vi "float_switch_check_debug.vi"(0 "Temperature Refnum":refnum<vi>, 1 "Heater Refnum":refnum<vi>, 2 "Abs Pressure Refnum":refnum<vi>, 3 "Abs Temperature Limit Refnum":refnum<vi>, 4 "Timeout Refnum":refnum<vi>, 5 "Abs Pressure Limit Refnum":refnum<vi>, 6 "STOP! Refnum":refnum<vi>, 7 "Pulse Generator Slide Refnum":refnum<vi>, 8 "Float Indicator Refnum":refnum<vi>[](array[refnum]), 9 "lines":tag[](array[tag])) -> ()   [LabVIEW 2015]
uses:
  <vilib>/DAQmx/create/channels.llb/DAQmx Create Channel (DI-Digital Input).vi
  <vilib>/DAQmx/read.llb/DAQmx Read (Digital 1D Bool NChan 1Samp 1Line).vi
panel:
  out "Stopwatch Elapsed":dbl
  out "Stopwatch Start":dbl
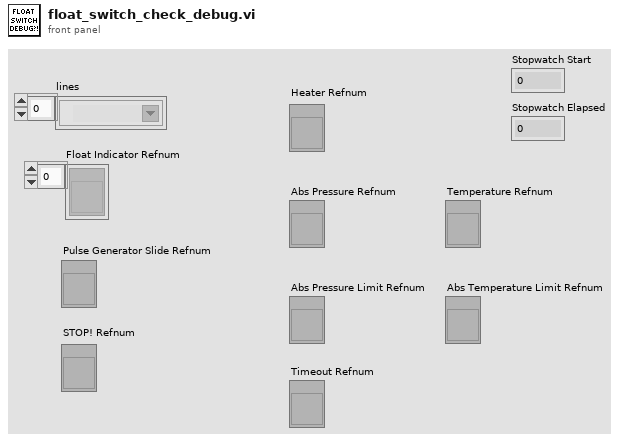
[diagram p1: front panel]
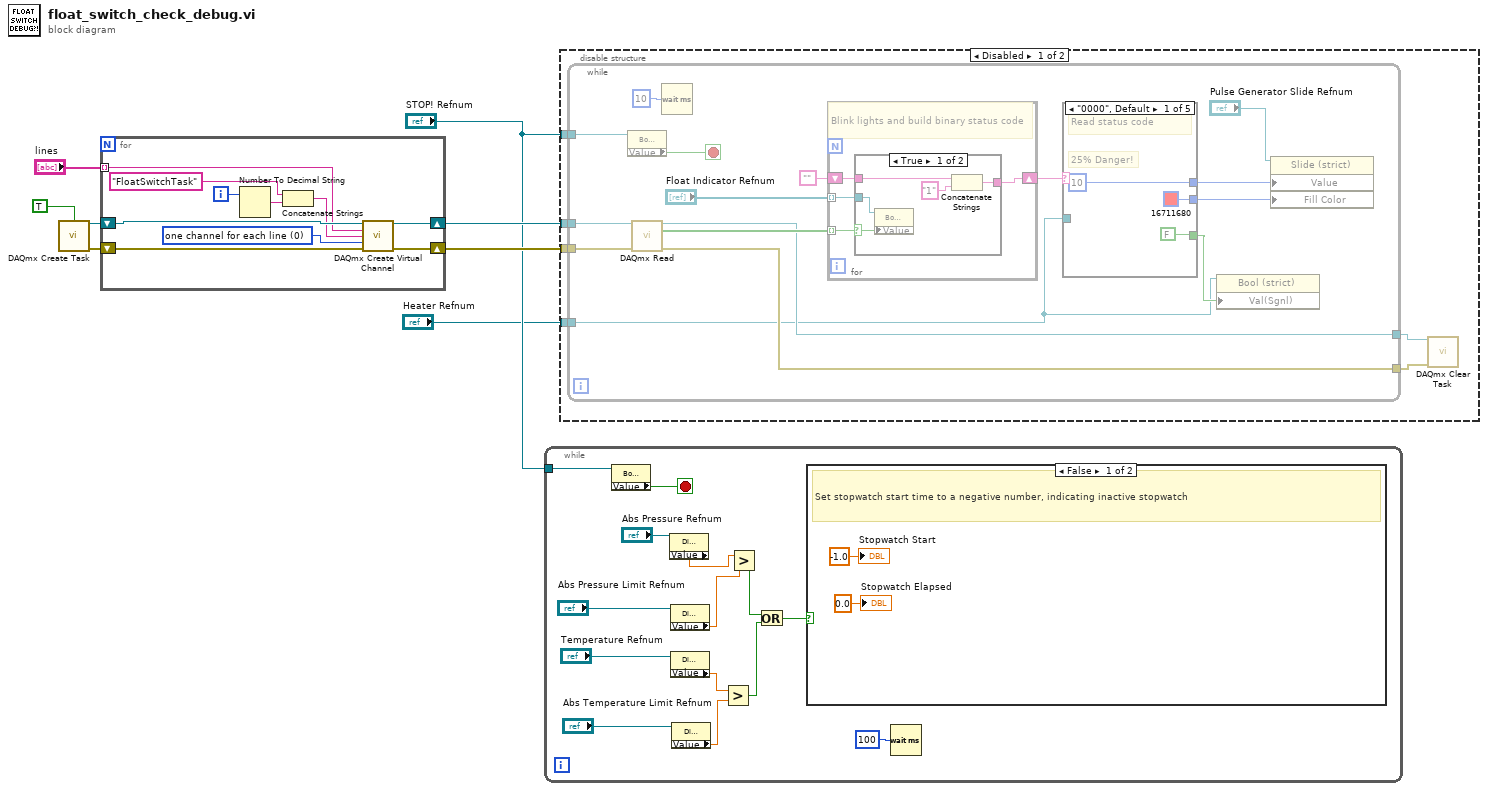
[diagram p0: block diagram]
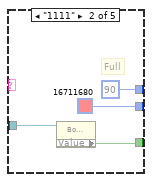
[diagram p2: hidden frame]
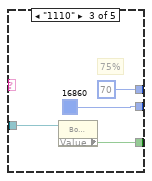
[diagram p3: hidden frame]
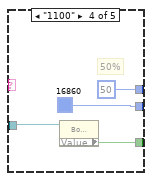
[diagram p4: hidden frame]
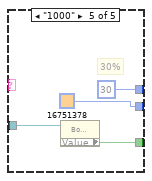
[diagram p5: hidden frame]
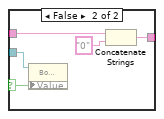
[diagram p6: hidden frame]
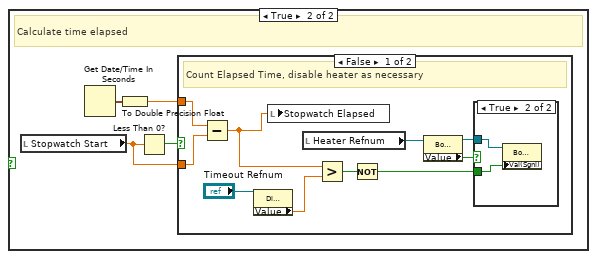
[diagram p8: hidden frame]
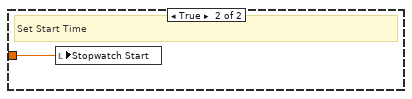
[diagram p10: hidden frame]
diagram:
  n1 = call <vilib>:"DAQmx Create Task.vi"("auto cleanup"=TRUE) -> ("task out"=w7:refnum<k21>, "error out"=w6:errorcluster)  [unwired: 13 in]
  n2 = for {
    shift-right: [w18] -> w5
    shift-left: w7 -> [w16]
    shift-right: [w17] -> w4
    shift-left: w6 -> [w15]
    tunnel: "lines" -> [w14] mode=indexing
    i -> [w9]
    w11 = 0 items=["one channel for each line", "one channel for all lines"] ("line grouping")
    n3 = Number To Decimal String(number=w9) -> (decimal integer string=w12:string)  [unwired: 1 in]
    n4 = Concatenate Strings("FloatSwitchTask" ("string"), w12) -> (w10:string)
    n5 = call-poly <vilib>:"DAQmx Create Virtual Channel.vi"("task in"=w16, "lines"=w14, "name to assign"=w10, "line grouping"=w11, "error in"=w15) -> ("task out"=w18:refnum<k21>, "error out"=w17:errorcluster)  [unwired: 9 in]
  }
  n6 = while {
    tunnel: "STOP! Refnum" -> [w31]
    stop <- w32 stop-if-true
    n7 = property class="Bool (strict)"(reference=w31) -> ("Value"=w32:bool)  [unwired: 1 in, 2 out]
    n8 = property class="DigNum (strict)"(reference="Abs Pressure Refnum") -> ("Value"=w20:dbl)  [unwired: 1 in, 2 out]
    n9 = property class="DigNum (strict)"(reference="Abs Pressure Limit Refnum") -> ("Value"=w19:dbl)  [unwired: 1 in, 2 out]
    n10 = property class="DigNum (strict)"(reference="Temperature Refnum") -> ("Value"=w25:dbl)  [unwired: 1 in, 2 out]
    n11 = property class="DigNum (strict)"(reference="Abs Temperature Limit Refnum") -> ("Value"=w24:dbl)  [unwired: 1 in, 2 out]
    n12 = Greater?(x=w25, y=w24) -> (0:w22:bool)
    n13 = Greater?(x=w20, y=w19) -> (0:w23:bool)
    n14 = Or(x=w23, y=w22) -> (x .or. y?=w21:bool)
    n15 = case shown="False" w21 {
      frame False {
        # "Set stopwatch start time to a negative number, indicating inactive stopwatch"
        "Stopwatch Start" <- -1.0 ("Stopwatch Start")
        "Stopwatch Elapsed" <- 0.0 ("Stopwatch Elapsed")
      }
      frame True {
        # "Calculate time elapsed"
        n16 = local read "Stopwatch Start"() -> (w35:dbl)
        n17 = Get Date/Time In Seconds() -> (seconds since 1Jan1904=w37:timestamp)
        n18 = To Double Precision Float(number=w37) -> (double precision float=w36:dbl)
        n19 = Less Than 0?(x=w35) -> (x < 0?=w38:bool)
        n20 = case shown="False" w38 {
          tunnel: w36 -> [w48 w51]
          tunnel: w35 -> [w47 _]
          frame False {
            # "Count Elapsed Time, disable heater as necessary"
            n21 = Subtract(x=w48, y=w47) -> (x-y=w43:dbl)
            n22 = property class="DigNum (strict)"(reference="Timeout Refnum") -> ("Value"=w45:dbl)  [unwired: 1 in, 2 out]
            n23 = local write "Stopwatch Elapsed"(w43) -> ()
            n24 = local read "Heater Refnum"() -> (w42:refnum<vi>)
            n25 = Greater?(x=w43, y=w45) -> (0:w44:bool)
            n26 = Not(x=w44) -> (.not. x?=w39:bool)
            n27 = property class="Bool (strict)"(reference=w42) -> (reference out=w40:refnum<vi>, "Value"=w41:bool)  [unwired: 1 in, 1 out]
            n28 = case shown="True" w41 {
              tunnel: w40 -> [_ w50]
              tunnel: w39 -> [_ w49]
              frame False {
              }
              frame True {
                n29 = property class="Bool (strict)"(reference=w50, "Val(Sgnl)"=w49) -> ()  [unwired: 1 in, 2 out]
              }
            }
          }
          frame True {
            # "Set Start Time"
            n30 = local write "Stopwatch Start"(w51) -> ()
          }
        }
      }
    }
    n31 = Wait (ms)(milliseconds to wait=u32 100) -> ()  [unwired: 1 out]
  }
  n32 = disable-structure shown="Disabled" {
    disable-tunnel: w5 -> [w57 _]
    disable-tunnel: w4 -> [w56 _]
    disable-tunnel: "STOP! Refnum" -> [w53 _]
    disable-tunnel: "Heater Refnum" -> [w52 _]
    frame Disabled {
      n33 = while {
        tunnel: w57 -> [w68]
        tunnel: w56 -> [w67]
        tunnel: w53 -> [w63]
        tunnel: [w60] -> w55
        tunnel: [w59] -> w54
        tunnel: w52 -> [w58]
        stop <- w62 stop-if-true
        n34 = property class="Bool (strict)"(reference=w63) -> ("Value"=w62:bool)  [unwired: 1 in, 2 out]
        n35 = call-poly <vilib>:"DAQmx Read.vi"("task/channels in"=w68, "error in"=w67) -> ("task out"=w60:refnum<k21>, "data"=w73:bool[], "error out"=w59:errorcluster)  [unwired: 11 in]
        n36 = Wait (ms)(milliseconds to wait=u32 10) -> ()  [unwired: 1 out]
        n37 = for {
          tunnel: w73 -> [w96] mode=indexing
          tunnel: "Float Indicator Refnum" -> [w95] mode=indexing
          shift-right: [w93] -> w71
          shift-left: "" -> [w94]
          # "Blink lights and build binary status code"
          n38 = case shown="True" w96 {
            selector: w96 -> [w100 w105]
            tunnel: w95 -> [w101 w106]
            tunnel: w94 -> [w99 w103]
            tunnel: [w97 w102] -> w93
            frame True {
              n39 = property class="Bool (strict)"(reference=w101, "Value"=w100) -> ()  [unwired: 1 in, 2 out]
              n40 = Concatenate Strings(w99, "1" ("string")) -> (w97:string)
            }
            frame False {
              n41 = property class="Bool (strict)"(reference=w106, "Value"=w105) -> ()  [unwired: 1 in, 2 out]
              n42 = Concatenate Strings(w103, "0" ("string")) -> (w102:string)
            }
          }
        }
        n43 = case shown="\"0000\", Default" w71 {
          tunnel: [u8 10 u8 90 u8 70 u8 50 u8 30] -> w70
          tunnel: [u32 16711680 u32 16711680 u32 16860 u32 16860 u32 16751378] -> w69
          tunnel: [FALSE w77 w81 w85 w89] -> w61
          tunnel: w58 -> [_ w78 w82 w86 w90]
          frame "0000", Default {
            # "25% Danger!"
            # "Read status code"
          }
          frame "1111" {
            # "Full"
            n44 = property class="Bool (strict)"(reference=w78) -> ("Value"=w77:bool)  [unwired: 1 in, 2 out]
          }
          frame "1110" {
            # "75%"
            n45 = property class="Bool (strict)"(reference=w82) -> ("Value"=w81:bool)  [unwired: 1 in, 2 out]
          }
          frame "1100" {
            # "50%"
            n46 = property class="Bool (strict)"(reference=w86) -> ("Value"=w85:bool)  [unwired: 1 in, 2 out]
          }
          frame "1000" {
            # "30%"
            n47 = property class="Bool (strict)"(reference=w90) -> ("Value"=w89:bool)  [unwired: 1 in, 2 out]
          }
        }
        n48 = property class="Bool (strict)"(reference=w58, "Val(Sgnl)"=w61) -> ()  [unwired: 1 in, 2 out]
        n49 = property class="Slide (strict)"(reference="Pulse Generator Slide Refnum", "Value"=w70, "Fill Color"=w69) -> ()  [unwired: 1 in, 2 out]
      }
      n50 = call <vilib>:"DAQmx Clear Task.vi"("task in"=w55, "error in"=w54) -> ()  [unwired: 13 in, 1 out]
    }
    frame Enabled {
    }
  }
